vi "toDateTimeString.vi"(6 "DateTimeFormatter (ISO8601)":refnum<class "DateTimeFormatter.lvclass">, 7 "UTC? (F)":bool, 9 "Fractional Second":dbl format="%#.6f", 10 "Epoch Time (s)":i64, 11 "Epoch":refnum<class "Epoch.lvclass">) -> (1 "Not a Timestamp?":bool, 2 "DateTime string":string, 3 "Epoch out":refnum<class "Epoch.lvclass">)   [LabVIEW 2018, in "Epoch.lvclass"]
uses:
  Epoch.lvclass
  formatter/DateTimeFormatter.lvclass
  formatter.iso8601/DateTime.ISO8601.lvclass
  C:/Users/Fujitsu/Documents/avril/Epoch Date & Time/formatter/DateTimeFormatter.lvclass
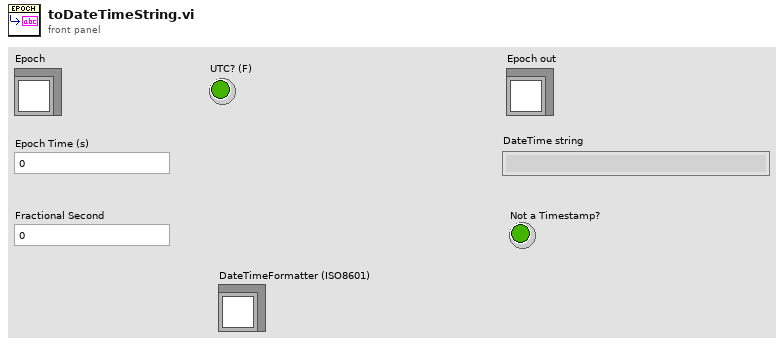
[diagram p1: front panel]
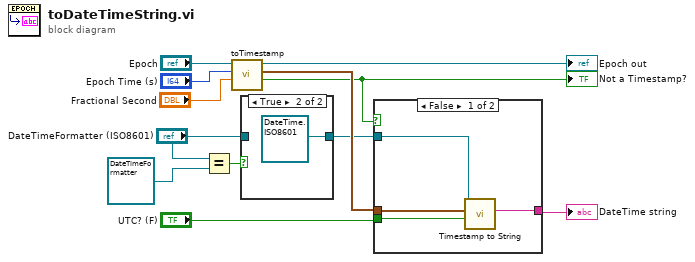
[diagram p0: block diagram]
diagram:
  n1 = Equal?(x="DateTimeFormatter (ISO8601)", y=refnum<class "DateTimeFormatter.lvclass"> refnum ("DateTimeFormatter.lvclass")) -> (x = y?=w5:bool)
  n2 = call-dynamic "toTimestamp.vi"("Fractional Second"="Fractional Second", "Epoch Time (s)"="Epoch Time (s)", "Epoch (Local)"="Epoch") -> ("Not a Timestamp?"=w2:bool, "Timestamp"=w7:timestamp, "Epoch (out)"=→"Epoch out":refnum<class "Epoch.lvclass">)  [unwired: 6 in]
  "Not a Timestamp?" <- w2
  n3 = case shown="True" w5 {
    tunnel: "DateTimeFormatter (ISO8601)" -> [w13 _]
    tunnel: [w13 refnum<class "DateTime.ISO8601.lvclass"> refnum ("Formatter.ISO8601.lvclass")] -> w3
    frame False {
    }
    frame True {
    }
  }
  n4 = case shown="False" w2 {
    tunnel: [w16 _] -> w8
    tunnel: w7 -> [w18 _]
    tunnel: "UTC? (F)" -> [w17 _]
    tunnel: w3 -> [w15 _]
    frame False {
      n5 = call "Timestamp to String.vi"("UTC? (F)"=w17, "Timestamp (now)"=w18, "DateTimeFormatter in"=w15) -> ("DateTime String"=w16:string)  [unwired: 6 in, 2 out]
    }
    frame True {
    }
  }
  "DateTime string" <- w8
